vi "PromVIEW Custom Collector Example.vi"   [LabVIEW 2020]
uses:
  src/registry/session/Registry Session.lvclass
  disk collector/Disk Collector.lvclass
types:
  T1 = typedef "Registry.lvlib/Registry Session.lvclass/Session Handle.ctl" = refnum<data-value>
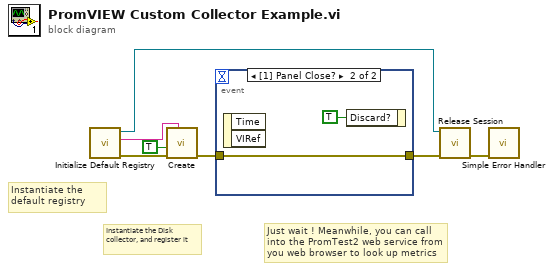
[diagram p0: block diagram]
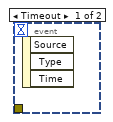
[diagram p2: hidden frame]
diagram:
  # "Just wait ! Meanwhile, you can call into the PromTest2 web service from you web browser to look up metrics"
  # "Instantiate the Disk collector, and register it"
  # "Instantiate the default registry"
  n1 = call "Initialize Default Registry.vi"() -> ("error out"=w7:errorcluster, "Registry Name"=w2:string, "Session Handle"=w5:T1)  [unwired: 9 in]
  n2 = call "Create.vi"("Registry Name"=w2, "error in (no error)"=w7, "Auto-Register? (T)"=TRUE) -> ("error out"=w6:errorcluster)  [unwired: 7 in, 1 out]
  n3 = event shown="[1] Panel Close?" {
    selector: _ -> [_ _]
    dyn-events: _ -> [_ _]
    timeout: _ -> [_ _]
    tunnel: w6 -> [_ w8]
    tunnel: [_ w8] -> w4
    event Timeout {
      n4 = event-data() -> ()  [unwired: 1 in, 3 out]
    }
    event Panel Close? {
      n5 = event-data() -> ()  [unwired: 1 in, 2 out]
      n6 = event-data("Discard?"=TRUE) -> ()  [unwired: 1 in, 1 out]
    }
  }
  n7 = call "Release Session.vi"("error in (no error)"=w4, "Session Handle"=w5) -> ("error out"=w3:errorcluster)  [unwired: 9 in]
  n8 = call <vilib>:"Simple Error Handler.vi"("error in (no error)"=w3) -> ()  [unwired: 4 in, 5 out]
